vi "Double FFT Measurement (Init Memory) test.vi"   [LabVIEW 2014]
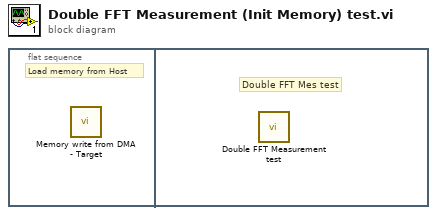
[diagram p0: block diagram]
diagram:
  n1 = flat-sequence {
    frame #0 {
      # "Load memory from Host"
      n2 = call "Memory write from DMA - Target.vi"() -> ()  [unwired: 12 in]
    }
    frame #1 {
      # "Double FFT Mes test"
      n3 = call "Double FFT Measurement test.vi"() -> ()  [unwired: 12 in]
    }
  }
